vi "Read.vi"(8 "error in (no error)":errorcluster, 11 "Boolean in":refnum<class "Const_Bool.lvclass">) -> (0 "error out":errorcluster, 2 "Boolean":bool, 3 "Boolean out":refnum<class "Const_Bool.lvclass">)   [LabVIEW 2021, in "Const_Bool.lvclass"]
uses:
  Const_Bool.lvclass
  Const_Bool.lvclass/Const_Bool.ctl
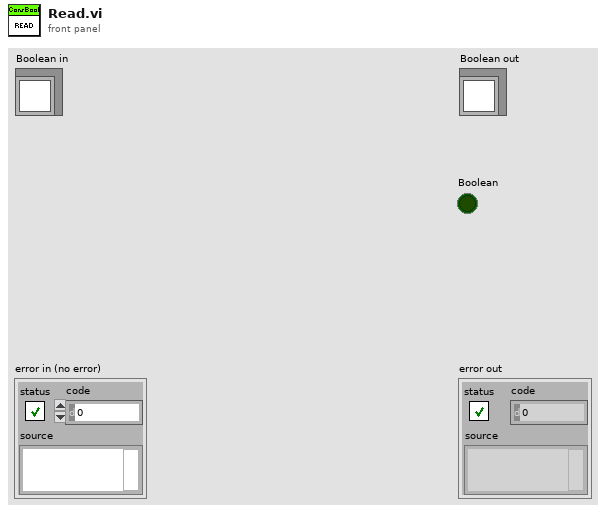
[diagram p1: front panel]
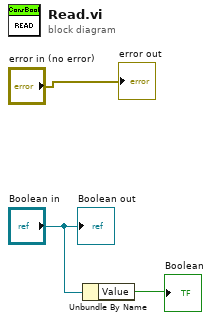
[diagram p0: block diagram]
diagram:
  n1 = Unbundle By Name("Boolean in") -> ("Value"=→"Boolean":bool)
  "error out" <- "error in (no error)"
  "Boolean out" <- "Boolean in"
